vi "AlazarReadU16.vi"(0 "Handle":u64, 1 "Channel":u32(ring)=1 items=["A"=1, "B"=2, "C"=4, "D"=8], 2 "Record":i32, 3 "Transfer Offset":i32, 4 "Transfer Length":u32, 5 "error in (no error)":errorcluster) -> (14 "Handle":u64, 15 "Buffer":u16[](array[numeric]), 18 "Return Code":u32, 19 "error out":errorcluster)   [LabVIEW 2018]
doc: "Read all or part of a record from an acquisition to on-board memory from on-board memory to a buffer in host memory. The record must be less than 2,147,483,648 samples long."
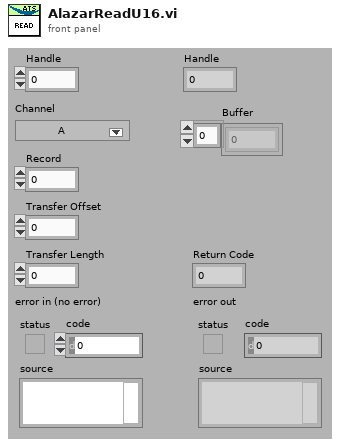
[diagram p1: front panel]
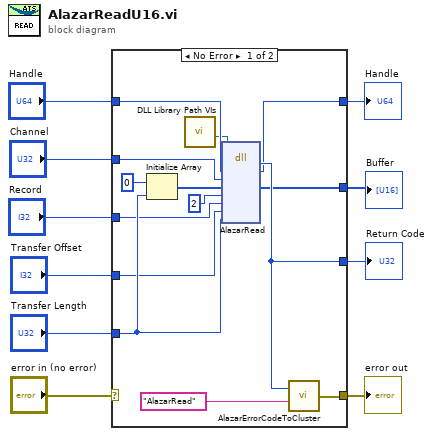
[diagram p0: block diagram]
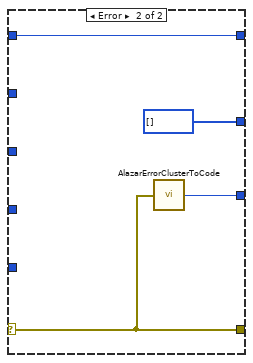
[diagram p2: hidden frame]
diagram:
  n1 = case shown="No Error" "error in (no error)" {
    selector: "error in (no error)" -> [_ w28]
    tunnel: [w21 w28] -> w9
    tunnel: [w23 w27] -> w8
    tunnel: "Handle" -> [w24 w26]
    tunnel: [w20 w26] -> w6
    tunnel: "Transfer Length" -> [w18 _]
    tunnel: "Transfer Offset" -> [w17 _]
    tunnel: "Record" -> [w16 _]
    tunnel: "Channel" -> [w13 _]
    tunnel: [w12 u16[] []] -> w1
    frame No Error {
      n2 = Initialize Array(u16 0, w18) -> (w15:u16[])
      n3 = call "DLL Library Path VIs.vi"() -> ("Alazar"=w11:path)  [unwired: 9 in, 2 out]
      n4 = dll-call lib="C:/Project/SerialSectOCT - FFT GPU/SerialSectOCT/Labview Software/DLL/ATSApi.dll" fn="AlazarRead"(path in=w11, "handle"=w24, "channelId"=w13, "buffer"=w15, "elementSize"=2, "record"=w16, "transferOffset"=w17, "transferLength"=w18) -> ("return type"=w23:u32, "handle"=w20:u64, "buffer"=w12:u16[])  [unwired: 7 in, 2 out]
      n5 = call "AlazarErrorCodeToCluster.vi"("Message"="AlazarRead", "Error Code"=w23) -> ("error out"=w21:errorcluster)
    }
    frame Error {
      n6 = call "AlazarErrorClusterToCode.vi"("error in (no error)"=w28) -> ("Error Code"=w27:u32)
    }
  }
  "Handle" <- w6
  "error out" <- w9
  "Return Code" <- w8
  "Buffer" <- w1
